vi "Gasflaschen Auswahl.vi"(8 "error in (no error)":errorcluster caption="Fehler (Eingang, kein Fehler)", 10 "Gasflaschen Liste gesamt":T1[](array[typedef]) {"Gasflasche"."Ablaufdatum" format="%<%d.%m.%Y>T"; "Komponenten"."Konzentration IST" format="%#.4f"; "Komponenten"."Genauigkeit" format="%#.1f"}, 11 "Ring (Eingang)":refnum<vi>) -> (0 "error out":errorcluster caption="Fehler (Ausgang)", 2 "Gasflaschen Liste gesamt out":T1[](array[typedef]) {"Gasflasche"."Ablaufdatum" format="%<%d.%m.%Y>T"; "Komponenten"."Konzentration IST" format="%#.4f"; "Komponenten"."Genauigkeit" format="%#.1f"}, 3 "Ring (Ausgang)":refnum<vi>)   [LabVIEW 2020, in "System Einstellungen V2.lvlib"]
uses:
  System Einstellungen V2.lvlib
  Gasflasche gesamt.ctl
  Gasflasche.ctl
  Traegergas.ctl
  Gasflaschenkomponente.ctl
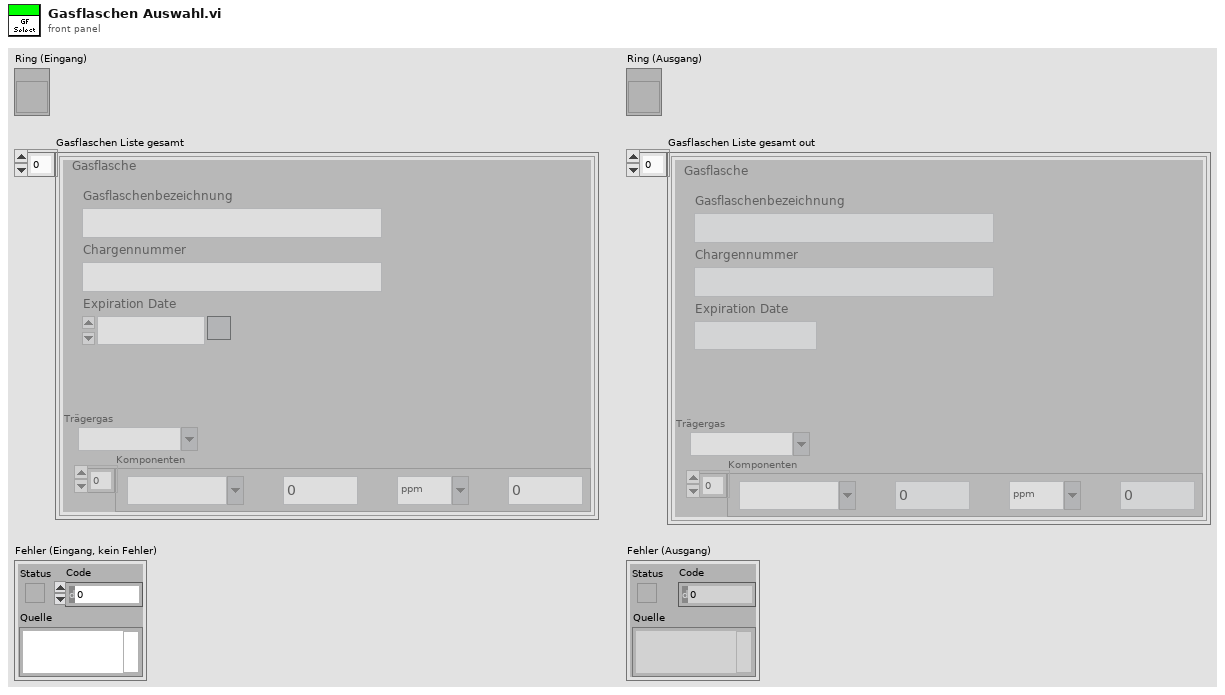
[diagram p1: front panel]
types:
  T1 = typedef "System Einstellungen V2.lvlib/Gasflasche gesamt.ctl" = cluster{"Gasflasche":T2, "Trägergas":T3, "Komponenten":T4[]}
  T2 = typedef "System Einstellungen V2.lvlib/Gasflasche.ctl" = cluster{"Gasname für die Auswahl":string, "Chargennummer":string, "Ablaufdatum":timestamp}
  T3 = typedef "System Einstellungen V2.lvlib/Traegergas.ctl" = string
  T4 = typedef "System Einstellungen V2.lvlib/Gasflaschenkomponente.ctl" = cluster{"Gasauswahl":string, "Konzentration IST":dbl, "Einheit":string, "Genauigkeit":dbl}
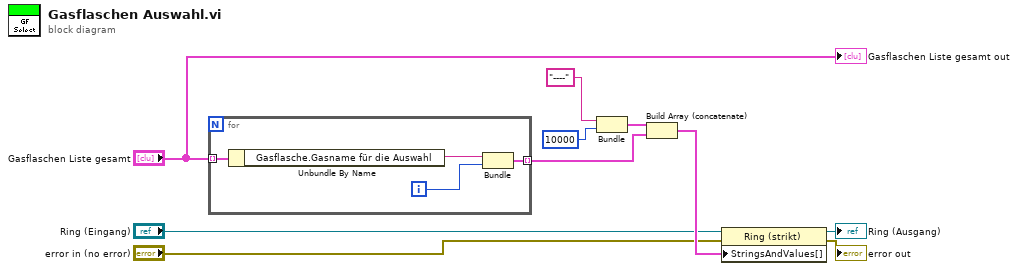
[diagram p0: block diagram]
diagram:
  n1 = for {
    tunnel: "Gasflaschen Liste gesamt" -> [w14] mode=indexing
    tunnel: [w12] -> w5 mode=indexing
    i -> [w13]
    n2 = Unbundle By Name(w14) -> ("Gasflasche.Gasname für die Auswahl"=w11:string)
    n3 = Bundle("Gasname für die Auswahl"=w11, w13) -> (w12:cluster{"Gasname für die Auswahl":string, i32})  [unwired: 1 in]
  }
  n4 = Bundle("----", 10000) -> (w6:cluster{string, i32})  [unwired: 1 in]
  n5 = Build Array (concatenate)(w6, w5) -> (w4:cluster{"Gasname für die Auswahl":string, i32}[])
  n6 = property on="Eigenschaftsknoten" class="Ring (strikt)"(reference="Ring (Eingang)", error in="error in (no error)", "StringsAndValues[]"=w4) -> (reference out=→"Ring (Ausgang)":refnum<vi>, error out=→"error out":errorcluster)
  "Gasflaschen Liste gesamt out" <- "Gasflaschen Liste gesamt"
